vi "Configure Curve Point.vi"(0 "VISA resource name":refnum<visa-resource-name>, 5 "Curve (21)":dbl=21.0, 7 "Index (1)":dbl=1.0, 9 "Units Value (0.00000)":dbl format="%.5f", 11 "error in (no error)":errorcluster, 12 "Temperature Value (0.0000)":dbl format="%.4f") -> (4 "VISA resource name out":refnum<visa-resource-name>, 15 "error out":errorcluster)   [LabVIEW 2020, in "Lake Shore 336.lvlib"]
doc: "This VI configures a curve point. Temperature response data of a calibrated sensor must be reduced to a table of breakpoints before entering it into the instrument. Each breakpoint consist of one value in sensor units and one temperature value in Kelvin. Linear interpolation is used by the instrument to calculate temperature between breakpoints. From 2 to 200 breakpoints can be entered as a curve.\n\nJonathan Billings, <billings@magnet.fsu.edu> NHMFL-FSU, March 2010\nCode added to properly encode six digit precision for <Units Value> and <Temperature Value>."
uses:
  Lake Shore 336.lvlib
  Instance           1 29Saved   Configure Curve Point .vi
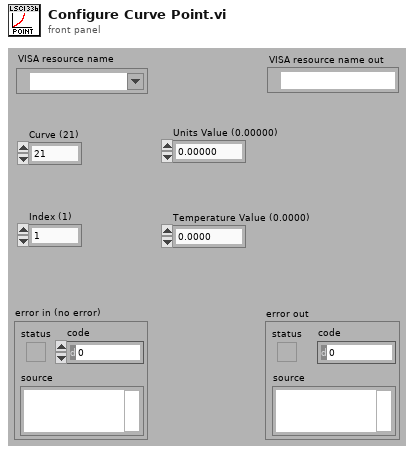
[diagram p1: front panel]
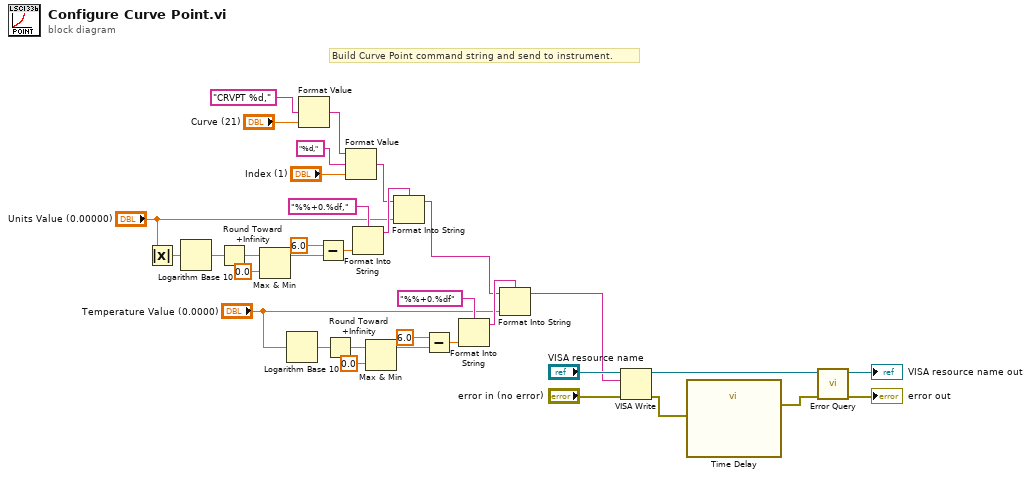
[diagram p0: block diagram]
diagram:
  # "Build Curve Point command string and send to instrument."
  n1 = Absolute Value(x="Units Value (0.00000)") -> (abs(x)=w14:dbl)
  n2 = Logarithm Base 10(1:w14) -> (0:w22:dbl)
  n3 = Round Toward +Infinity(x=w22) -> (ceil(x): smallest int >= x=w21:dbl)
  n4 = Max & Min(x=w21, y=0.0) -> (max(x,y)=w19:dbl)  [unwired: 1 out]
  n5 = Logarithm Base 10(1:"Temperature Value (0.0000)") -> (0:w11:dbl)
  n6 = Format Value(format string="CRVPT %d,", value (0)="Curve (21)") -> (output string=w26:string)  [unwired: 1 in]
  n7 = Subtract(x=6.0, y=w19) -> (x-y=w18:dbl)
  n8 = Round Toward +Infinity(x=w11) -> (ceil(x): smallest int >= x=w10:dbl)
  n9 = Format Value(string ("")=w26, format string="%d,", value (0)="Index (1)") -> (output string=w12:string)
  n10 = Format Into String(format string="%%+0.%df,", w18) -> (resulting string=w16:string)  [unwired: 2 in, 1 out]
  n11 = Max & Min(x=w10, y=0.0) -> (max(x,y)=w8:dbl)  [unwired: 1 out]
  n12 = Format Into String(format string=w16, initial string=w12, "Units Value (0.00000)") -> (resulting string=w3:string)  [unwired: 1 in, 1 out]
  n13 = Subtract(x=6.0, y=w8) -> (x-y=w7:dbl)
  n14 = Format Into String(format string="%%+0.%df", w7) -> (resulting string=w5:string)  [unwired: 2 in, 1 out]
  n15 = Format Into String(format string=w5, initial string=w3, "Temperature Value (0.0000)") -> (resulting string=w1:string)  [unwired: 1 in, 1 out]
  n16 = VISA Write(VISA resource name="VISA resource name", write buffer=w1, error in (no error)="error in (no error)") -> (VISA resource name out=w32:refnum<visa-resource-name>, error out=w24:errorcluster)  [unwired: 1 out]
  n17 = call "Time Delay"("error in (no error)"=w24) -> ("error out"=w23:errorcluster)  [unwired: 10 in]
  n18 = call "Error Query.vi"("error in (no error)"=w23, "VISA resource name"=w32) -> ("error out"=→"error out":errorcluster, "VISA resource name out"=→"VISA resource name out":refnum<visa-resource-name>)  [unwired: 7 in, 1 out]
